vi "Remove Topic Subscriber.vi"(8 "error in (no error)":errorcluster, 10 "Subscription Policy":T1, 11 "Topic in":refnum<class "Topic.lvclass">) -> (0 "error out":errorcluster, 3 "Topic out":refnum<class "Topic.lvclass">)   [LabVIEW 2018, in "MVA Framework.lvlib" / "Mediator.lvlib" / "Topic.lvclass"]
doc: "删除主题订阅者"
uses:
  Topic.lvclass
  IMediator/ISubscriptionPolicy/ISubscriptionPolicy.lvclass
  IMediator/ISubscriptionPolicy/ISubscriptionPolicy Reference.ctl
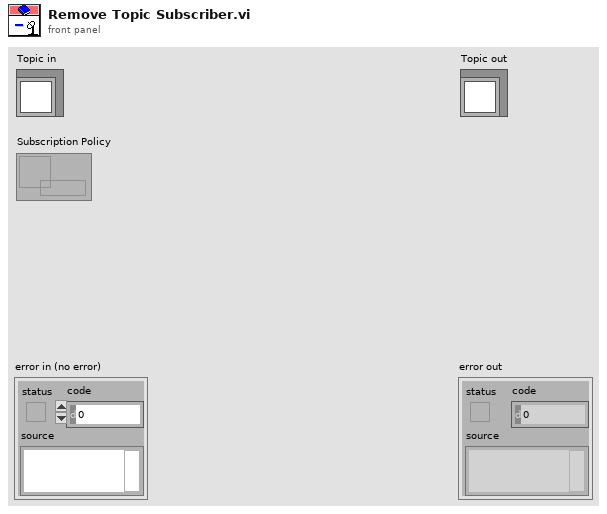
[diagram p1: front panel]
types:
  T1 = typedef "MVA Framework.lvlib/IMediator.lvlib/ISubscriptionPolicy.lvclass/ISubscriptionPolicy Reference.ctl" = refnum<data-value>
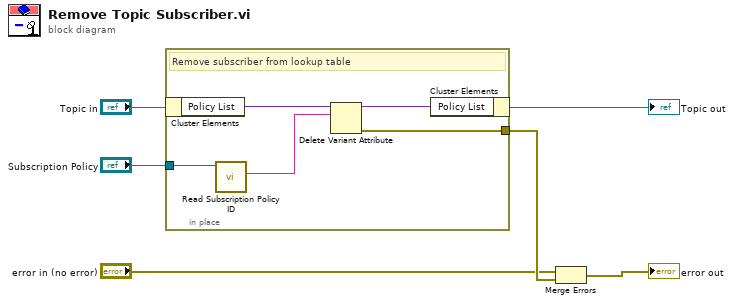
[diagram p0: block diagram]
diagram:
  n1 = in-place {
    in-place-border: [w10] -> w6
    in-place-border: "Subscription Policy" -> [w7]
    # "Remove subscriber from lookup table"
    n2 = in-place-cluster #1("Topic in") -> ("Policy List"=w9:variant)
    n3 = call "Read Subscription Policy ID.vi"("SubscriptionPolicy"=w7) -> ("Policy ID"=w8:string)  [unwired: 10 in]
    n4 = Delete Variant Attribute(6:w8, 7:w9) -> (0:w10:errorcluster, 3:w11:variant)  [unwired: 1 in, 1 out]
    n5 = in-place-cluster #1("Policy List"=w11) -> (→"Topic out":refnum<class "Topic.lvclass">)
  }
  n6 = Merge Errors("error in (no error)", w6) -> (→"error out":errorcluster)
